vi "Video Cam Processor Create.vi"(4 "Num Threads (-1: CPU count)":i32=-1, 5 "Identifier":string, 6 "Depth History Size (10)":i32=10, 7 "Open? (T)":bool=TRUE, 8 "error in (no error)":errorcluster, 9 "Sensor Index (0)":i32, 10 "Device Index (0)":i32, 11 "Video Processor in":refnum<class "Video Cam Processor.lvclass">) -> (0 "error out":errorcluster, 3 "Video Processor out":refnum<class "Video Cam Processor.lvclass">)   [LabVIEW 2018, in "Video Cam Processor.lvclass"]
uses:
  Video Cam Processor.lvclass
  C:/Users/aaron.jencks/Documents/GitHub/emerson_seed_object_detection/LabVIEW/Projects/Paul's Video Viewer/Classes/Video Processor/Video Processor.lvclass
  C:/Users/aaron.jencks/Documents/GitHub/emerson_seed_object_detection/LabVIEW/Projects/Paul's Video Viewer/Classes/Realsense Cam Video File Wrapper/Realsense Cam File Wrapper.lvclass
  Realsense Cam Video File Wrapper/Realsense Cam File Wrapper.lvclass
  Video Processor/Video Processor.lvclass
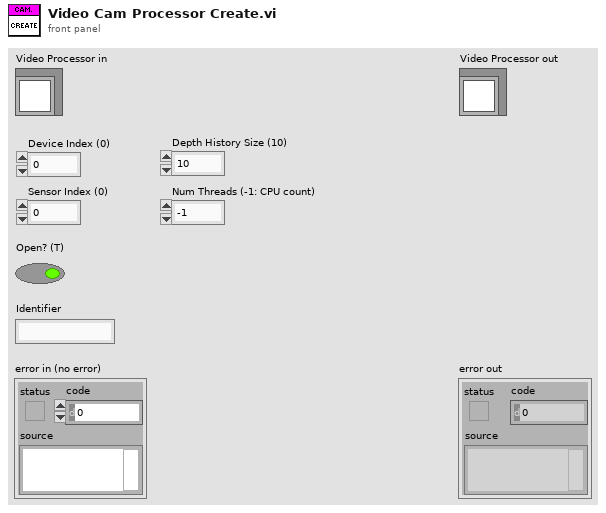
[diagram p1: front panel]
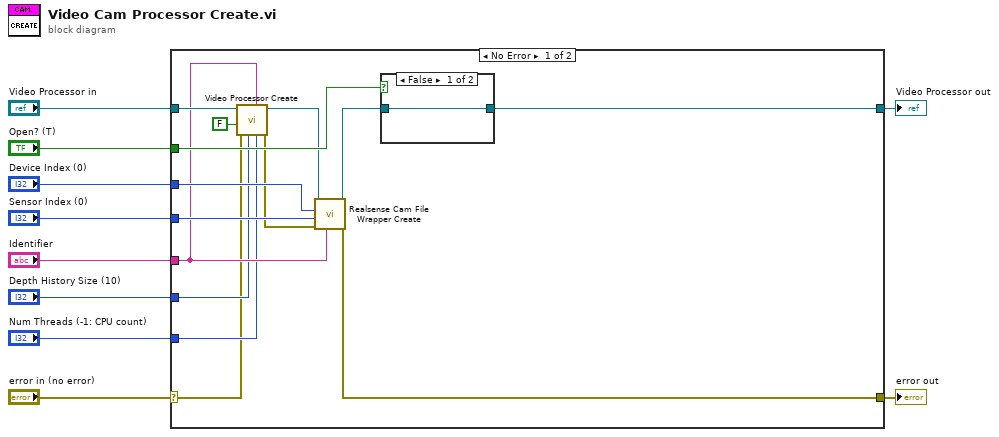
[diagram p0: block diagram]
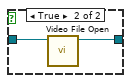
[diagram p2: hidden frame]
diagram:
  n1 = case shown="No Error" "error in (no error)" {
    selector: "error in (no error)" -> [w13 w29]
    tunnel: [w11 w29] -> w9
    tunnel: [w14 w28] -> w7
    tunnel: "Video Processor in" -> [w20 w28]
    tunnel: "Identifier" -> [w18 _]
    tunnel: "Depth History Size (10)" -> [w16 _]
    tunnel: "Num Threads (-1: CPU count)" -> [w15 _]
    tunnel: "Open? (T)" -> [w21 _]
    tunnel: "Device Index (0)" -> [w24 _]
    tunnel: "Sensor Index (0)" -> [w23 _]
    frame No Error {
      n2 = call "Video Processor Create.vi"("Num Threads (-1: CPU count)"=w15, "Identifier"=w18, "Depth History Size (10)"=w16, "error in (no error)"=w13, "Open File? (T)"=FALSE, "Video Processor in"=w20) -> ("error out"=w12:errorcluster, "Video Processor out"=w19:refnum<class "Video Cam Processor.lvclass">)  [unwired: 4 in]
      n3 = call "Realsense Cam File Wrapper Create.vi"("Identifier"=w18, "error in (no error)"=w12, "Sensor Index (0)"=w23, "Device Index (0)"=w24, "Realsense Cam File Wrapper in"=w19) -> ("error out"=w11:errorcluster, "Realsense Cam File Wrapper out"=w22:refnum<class "Video Cam Processor.lvclass">)  [unwired: 5 in]
      n4 = case shown="False" w21 {
        tunnel: w22 -> [w25 w27]
        tunnel: [w25 w26] -> w14
        frame False {
        }
        frame True {
          n5 = call-dynamic "Video File Open.vi"("Realsense Cam File Wrapper in"=w27) -> ("Realsense Cam File Wrapper out"=w26:refnum<class "Video Cam Processor.lvclass">)  [unwired: 9 in, 1 out]
        }
      }
    }
    frame Error {
    }
  }
  "error out" <- w9
  "Video Processor out" <- w7
